vi "Function.vi"(8 "error in (no error)":errorcluster, 10 "Value":dbl, 11 "Two Terminal in":refnum<class "Increment_CPLX_DBL.lvclass">) -> (0 "error out":errorcluster, 2 "Result":dbl, 3 "Two Terminal out":refnum<class "Increment_CPLX_DBL.lvclass">)   [LabVIEW 2021, in "Increment_CPLX_DBL.lvclass"]
uses:
  Increment_CPLX_DBL.lvclass
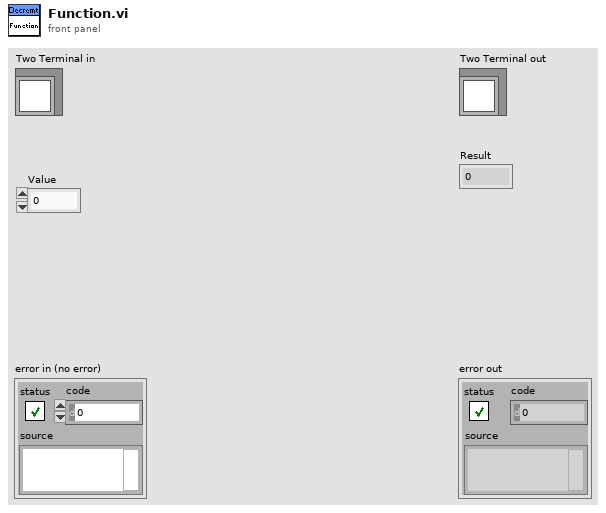
[diagram p1: front panel]
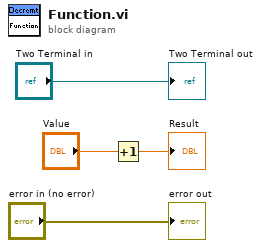
[diagram p0: block diagram]
diagram:
  n1 = Increment(x="Value") -> (x+1=→"Result":dbl)
  "error out" <- "error in (no error)"
  "Two Terminal out" <- "Two Terminal in"
